vi "FPGA Debug.vi"() -> ()   [LabVIEW 2018]
uses:
  <vilib>/rvi/Emulation/niFpgaGetClockAttributes.vi
  <vilib>/rvi/Emulation/niFpgaSctlEmulationGetInTimedLoop.vi
  <vilib>/rvi/Emulation/niFpgaEmulationReportErrorSimple.vi
  <vilib>/rvi/eio/common/nirviEmuTemplateMethod_errors.vi
  <vilib>/rvi/Emulation/niFpgaCriticalErrorInLSC.vi
  <vilib>/eio/EIONode/EIONode.xnode
  <vilib>/eio/EIOMethodNode/EIOMethodNode.xnode
panel:
  in  "Voltage Out":fxp<+/-,20,5>[](array[numeric])=[0.0, 0.0, 0.0, 0.0]
  in  "Digital Out":bool[](array[boolean])=[FALSE, FALSE, FALSE, FALSE, FALSE, FALSE, FALSE, FALSE]
  out "Digital In":bool[](array[boolean])
  out "LS AI":fxp<+/-,26,5>[](array[numeric])
  out "Current In":fxp<+/-,21,-4>[](array[numeric])
  out "HS AI":fxp<+/-,24,-4>[](array[numeric])
  out "RTDs":fxp<+/-,24,10>[](array[numeric])
  out "Thermocouples":fxp<+/-,24,-2>[](array[numeric])
  # "Ball valve control"
  # "butterfly valve control"
  # "enable something else"
  # "enable motor"
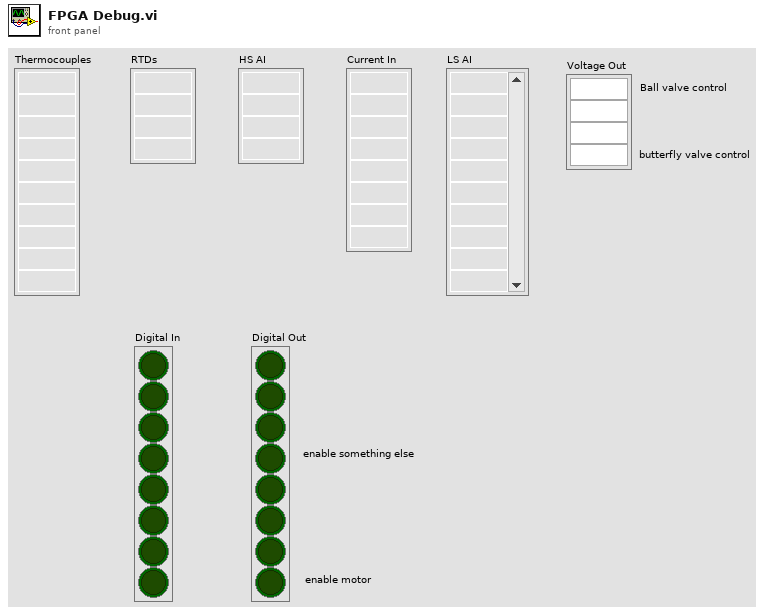
[diagram p1: front panel]
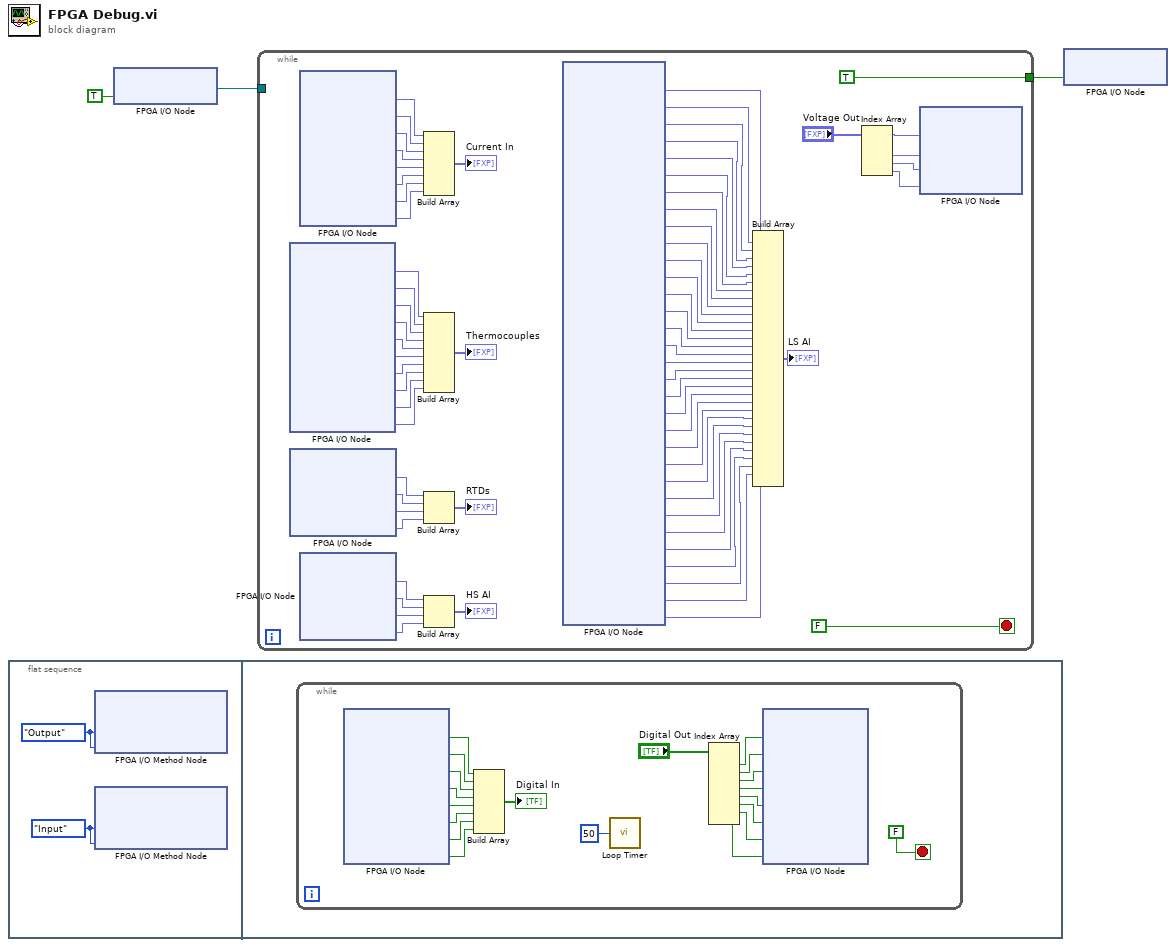
[diagram p0: block diagram]
diagram:
  n1 = flat-sequence {
    frame #0 {
      w5 = enum8{"No Change", "Input", "Output"}."Input" ("DIO 7:4")
      w4 = enum8{"No Change", "Input", "Output"}."Output" ("DIO 7:4")
      n2 = xnode "FPGA I/O Method Node"("DIO 7:4"=w4, "DIO 3:0"=w4) -> ()  [unwired: 1 in, 1 out]
      n3 = xnode "FPGA I/O Method Node"("DIO 7:4"=w5, "DIO 3:0"=w5) -> ()  [unwired: 1 in, 1 out]
    }
    frame #1 {
      n4 = while {
        stop <- FALSE stop-if-true
        n5 = xnode "FPGA I/O Node"() -> ("Mod7/DIO0"=w25:bool, "Mod7/DIO1"=w24:bool, "Mod7/DIO2"=w23:bool, "Mod7/DIO3"=w22:bool, "Mod7/DIO4"=w21:bool, "Mod7/DIO5"=w20:bool, "Mod7/DIO6"=w19:bool, "Mod7/DIO7"=w18:bool)  [unwired: 8 in, 8 out]
        n6 = Build Array(w25, w24, w23, w22, w21, w20, w19, w18) -> (→"Digital In":bool[])
        n7 = call "Loop Timer"("Count(mSec)"=u32 50) -> ()  [unwired: 1 out]
        n8 = Index Array(array="Digital Out") -> (element #1=w16:bool, element #2=w15:bool, element #3=w14:bool, element #4=w13:bool, element #5=w12:bool, element #6=w11:bool, element #7=w10:bool, element #8=w9:bool)  [unwired: 8 in]
        n9 = xnode "FPGA I/O Node"("Mod8/DIO0"=w16, "Mod8/DIO1"=w15, "Mod8/DIO2"=w14, "Mod8/DIO3"=w13, "Mod8/DIO4"=w12, "Mod8/DIO5"=w11, "Mod8/DIO6"=w10, "Mod8/DIO7"=w9) -> ()  [unwired: 8 in, 8 out]
      }
    }
  }
  n10 = xnode "FPGA I/O Node"("Mod3/Start"=TRUE) -> ("FPGA I/O Out"=w2:refnum<k21>)  [unwired: 1 in]
  n11 = while {
    tunnel: [TRUE ("Mod3/Start")] -> w1
    tunnel: w2 -> [_]
    stop <- FALSE stop-if-true
    n12 = xnode "FPGA I/O Node"() -> ("Mod1/TC0"=w94:fxp<+/-,24,-2>, "Mod1/TC1"=w93:fxp<+/-,24,-2>, "Mod1/TC2"=w92:fxp<+/-,24,-2>, "Mod1/TC3"=w91:fxp<+/-,24,-2>, "Mod1/TC4"=w90:fxp<+/-,24,-2>, "Mod1/TC5"=w88:fxp<+/-,24,-2>, "Mod1/TC6"=w89:fxp<+/-,24,-2>, "Mod1/TC7"=w87:fxp<+/-,24,-2>, "Mod1/CJC0"=w86:fxp<+/-,24,-2>, "Mod1/CJC1"=w85:fxp<+/-,24,-2>)  [unwired: 10 in, 10 out]
    n13 = xnode "FPGA I/O Node"() -> ("Mod2/RTD0"=w83:fxp<+/-,24,10>, "Mod2/RTD1"=w82:fxp<+/-,24,10>, "Mod2/RTD2"=w81:fxp<+/-,24,10>, "Mod2/RTD3"=w80:fxp<+/-,24,10>)  [unwired: 4 in, 4 out]
    n14 = xnode "FPGA I/O Node"() -> ("Mod4/AI0"=w73:fxp<+/-,21,-4>, "Mod4/AI1"=w72:fxp<+/-,21,-4>, "Mod4/AI2"=w71:fxp<+/-,21,-4>, "Mod4/AI3"=w70:fxp<+/-,21,-4>, "Mod4/AI4"=w69:fxp<+/-,21,-4>, "Mod4/AI5"=w68:fxp<+/-,21,-4>, "Mod4/AI6"=w67:fxp<+/-,21,-4>, "Mod4/AI7"=w66:fxp<+/-,21,-4>)  [unwired: 8 in, 8 out]
    n15 = xnode "FPGA I/O Node"() -> ("Mod3/AI0"=w78:fxp<+/-,24,-4>, "Mod3/AI1"=w77:fxp<+/-,24,-4>, "Mod3/AI2"=w76:fxp<+/-,24,-4>, "Mod3/AI3"=w75:fxp<+/-,24,-4>)  [unwired: 4 in, 4 out]
    n16 = Build Array(w73, w72, w71, w70, w69, w68, w67, w66) -> (→"Current In":fxp<+/-,21,-4>[])
    n17 = Build Array(w94, w93, w92, w91, w90, w88, w89, w87, w86, w85) -> (→"Thermocouples":fxp<+/-,24,-2>[])
    n18 = Build Array(w83, w82, w81, w80) -> (→"RTDs":fxp<+/-,24,10>[])
    n19 = Build Array(w78, w77, w76, w75) -> (→"HS AI":fxp<+/-,24,-4>[])
    n20 = xnode "FPGA I/O Node"() -> ("Mod5/AI0"=w63:fxp<+/-,26,5>, "Mod5/AI1"=w62:fxp<+/-,26,5>, "Mod5/AI2"=w61:fxp<+/-,26,5>, "Mod5/AI3"=w60:fxp<+/-,26,5>, "Mod5/AI4"=w59:fxp<+/-,26,5>, "Mod5/AI5"=w58:fxp<+/-,26,5>, "Mod5/AI6"=w57:fxp<+/-,26,5>, "Mod5/AI7"=w56:fxp<+/-,26,5>, "Mod5/AI8"=w32:fxp<+/-,26,5>, "Mod5/AI9"=w33:fxp<+/-,26,5>, "Mod5/AI10"=w34:fxp<+/-,26,5>, "Mod5/AI11"=w35:fxp<+/-,26,5>, "Mod5/AI12"=w36:fxp<+/-,26,5>, "Mod5/AI13"=w37:fxp<+/-,26,5>, "Mod5/AI14"=w38:fxp<+/-,26,5>, "Mod5/AI15"=w39:fxp<+/-,26,5>, "Mod5/AI16"=w40:fxp<+/-,26,5>, "Mod5/AI17"=w41:fxp<+/-,26,5>, "Mod5/AI18"=w42:fxp<+/-,26,5>, "Mod5/AI19"=w43:fxp<+/-,26,5>, "Mod5/AI20"=w44:fxp<+/-,26,5>, "Mod5/AI21"=w45:fxp<+/-,26,5>, "Mod5/AI22"=w46:fxp<+/-,26,5>, "Mod5/AI23"=w47:fxp<+/-,26,5>, "Mod5/AI24"=w48:fxp<+/-,26,5>, "Mod5/AI25"=w49:fxp<+/-,26,5>, "Mod5/AI26"=w50:fxp<+/-,26,5>, "Mod5/AI27"=w51:fxp<+/-,26,5>, "Mod5/AI28"=w52:fxp<+/-,26,5>, "Mod5/AI29"=w53:fxp<+/-,26,5>, "Mod5/AI30"=w54:fxp<+/-,26,5>, "Mod5/AI31"=w55:fxp<+/-,26,5>)  [unwired: 32 in, 32 out]
    n21 = Build Array(w63, w62, w61, w60, w59, w58, w57, w56, w32, w33, w34, w35, w36, w37, w38, w39, w40, w41, w42, w43, w44, w45, w46, w47, w48, w49, w50, w51, w52, w53, w54, w55) -> (→"LS AI":fxp<+/-,26,5>[])
    n22 = Index Array(array="Voltage Out") -> (element #1=w29:fxp<+/-,20,5>, element #2=w28:fxp<+/-,20,5>, element #3=w27:fxp<+/-,20,5>, element #4=w26:fxp<+/-,20,5>)  [unwired: 4 in]
    n23 = xnode "FPGA I/O Node"("Mod6/AO0"=w29, "Mod6/AO1"=w28, "Mod6/AO2"=w27, "Mod6/AO3"=w26) -> ()  [unwired: 4 in, 4 out]
  }
  n24 = xnode "FPGA I/O Node"("Mod3/Stop"=w1) -> ()  [unwired: 1 in, 1 out]
